vi "LHF.DB.Mongo.Collection.JSON.Insert.vi"(6 "Extract _id (T)":bool=TRUE, 7 "JSON document":string, 8 "error in (no error)":errorcluster, 9 "_id":string, 10 "Collection":string, 11 "LHF.DB.Mongo":refnum<class "LHF.DB.Mongo.lvclass">) -> (0 "error out":errorcluster, 1 "_id":string, 2 "Ok":bool, 3 "LHF.DB.Mongo out":refnum<class "LHF.DB.Mongo.lvclass">)   [LabVIEW 2013, in "LHF.DB.Mongo.lvclass"]
doc: "Wire cluster to Document Variant terminal. Cluster element names will be used as field names."
uses:
  LHF.DB.Mongo.lvclass
  C:/Users/Ricardo/Desktop/Projetos/LabVIEW-MongoDB/src/Driver/MongoDB.Bson.dll
  Driver/MongoDB.Bson.dll
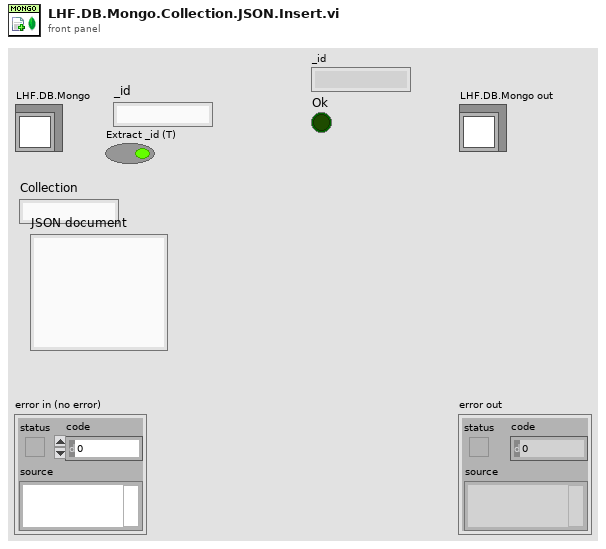
[diagram p1: front panel]
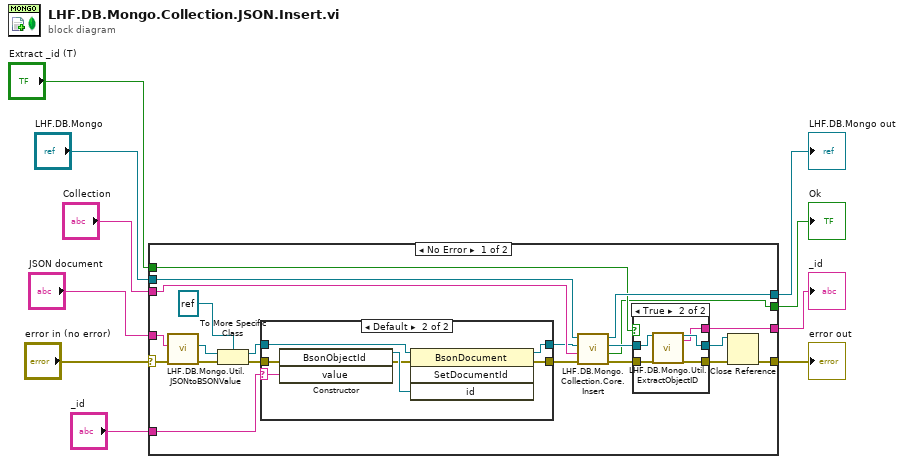
[diagram p0: block diagram]
diagram:
  n1 = case shown="No Error" "error in (no error)" {
    selector: "error in (no error)" -> [w14 w49]
    tunnel: [w15 w49] -> w9
    tunnel: [w30 w48] -> w7
    tunnel: "LHF.DB.Mongo" -> [w23 w48]
    tunnel: "JSON document" -> [w11 _]
    tunnel: "Collection" -> [w31 _]
    tunnel: [w16 _] -> w4
    tunnel: "_id" -> [w29 _]
    tunnel: "Extract _id (T)" -> [w25 _]
    tunnel: [w24 _] -> w1
    frame No Error {
      n2 = call "LHF.DB.Mongo.Util.JSONtoBSONValue.vi"("error in (no error)"=w14, "JSON data"=w11) -> ("error out"=w13:errorcluster, "BsonValue"=w12:refnum<k24>)  [unwired: 8 in]
      n3 = To More Specific Class(target class=refnum<k24> refnum ("BsonDocument"), reference=w12, error in=w13) -> (specific class reference=w21:refnum<k24>, error out=w19:errorcluster)
      n4 = case shown="Default" w29 {
        selector: w29 -> [_ w44]
        tunnel: w21 -> [w40 w47]
        tunnel: [w40 w46] -> w22
        tunnel: w19 -> [w39 w43]
        tunnel: [w39 w41] -> w28
        frame "" {
        }
        frame Default {
          n5 = constructor class="BsonObjectId"(error in=w43, "value"=w44) -> (reference out=w45:refnum<k24>, error out=w42:errorcluster)  [unwired: 2 in, 2 out]
          n6 = invoke class="BsonDocument" method="SetDocumentId"(reference=w47, error in=w42, "id"=w45) -> (reference out=w46:refnum<k24>, error out=w41:errorcluster)  [unwired: 1 in, 2 out]
        }
      }
      n7 = call "LHF.DB.Mongo.Collection.Core.Insert.vi"("error in (no error)"=w28, "collectionName"=w31, "BsonDocument"=w22, "LHF.DB.Mongo in"=w23) -> ("error out"=w26:errorcluster, "Ok"=w16:bool, "BsonDocument out"=w27:refnum<k24>, "LHF.DB.Mongo out"=w30:refnum<class "LHF.DB.Mongo.lvclass">)  [unwired: 4 in]
      n8 = case shown="True" w25 {
        tunnel: w27 -> [w32 w38]
        tunnel: [w32 w37] -> w18
        tunnel: w26 -> [w33 w36]
        tunnel: [w33 w35] -> w17
        tunnel: [_ w34] -> w24
        frame False {
        }
        frame True {
          n9 = call "LHF.DB.Mongo.Util.ExtractObjectID.vi"("BsonDocument Refnum in"=w38, "error in (no error)"=w36) -> ("BsonDocument Refnum out"=w37:refnum<k24>, "_id"=w34:string, "error out"=w35:errorcluster)  [unwired: 15 in]
        }
      }
      n10 = Close Reference(reference=w18, error in (no error)=w17) -> (error out=w15:errorcluster)
    }
    frame Error {
    }
  }
  "error out" <- w9
  "LHF.DB.Mongo out" <- w7
  "_id" <- w1
  "Ok" <- w4
